vi "Read Discrete Inputs.vi"(8 "error in":errorcluster, 9 "number of inputs":u16, 10 "starting address":u16, 11 "Modbus master in":refnum<class "Modbus Master.lvclass">) -> (0 "error out":errorcluster, 2 "discrete inputs":bool[](array[boolean]), 3 "Modbus master out":refnum<class "Modbus Master.lvclass">)   [LabVIEW 2012, in "Modbus Master.lvclass"]
doc: "Reads <B>number of inputs</B> discrete inputs starting at <B>starting address</B> from the device."
uses:
  Modbus Master.lvclass
  Modbus API.lvclass/Modbus API.ctl
  Modbus Master.lvclass/Modbus Master.ctl
  Transmission Data Unit/Transmission Data Unit.lvclass
  Modbus API.lvclass
  Master Function Definition/Master Function Definition.lvclass
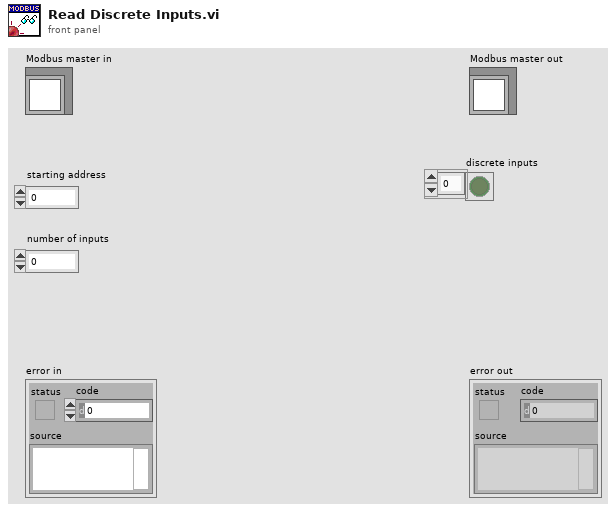
[diagram p1: front panel]
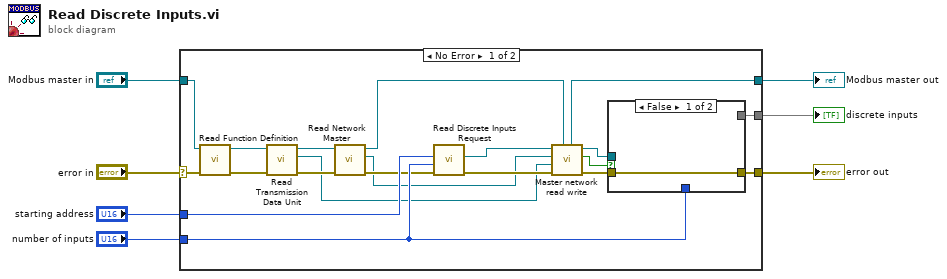
[diagram p0: block diagram]
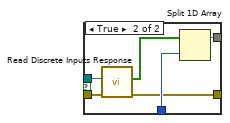
[diagram p2: hidden frame]
diagram:
  n1 = case shown="No Error" "error in" {
    selector: "error in" -> [w14 w35]
    tunnel: "Modbus master in" -> [w11 w36]
    tunnel: [w19 w36] -> w6
    tunnel: [w20 w35] -> w5
    tunnel: [w25 _] -> w3
    tunnel: "number of inputs" -> [w24 _]
    tunnel: "starting address" -> [w26 _]
    frame No Error {
      n2 = call "Read Function Definition.vi"("error in"=w14, "Modbus master in"=w11) -> ("error out"=w17:errorcluster, "Modbus master out"=w16:refnum<class "Modbus Master.lvclass">)  [unwired: 7 in, 1 out]
      n3 = call "Read Transmission Data Unit.vi"("error in"=w17, "Modbus instance in"=w16) -> ("error out"=w15:errorcluster, "transmission data unit"=w10:refnum<class "Transmission Data Unit.lvclass">, "Modbus instance out"=w18:refnum<class "Modbus Master.lvclass">)  [unwired: 7 in]
      n4 = call "Read Network Master.vi"("error in"=w15, "Modbus master in"=w18) -> ("error out"=w13:errorcluster, "network master"=w9:refnum<class "Network Master.lvclass">, "Modbus master out"=w12:refnum<class "Modbus Master.lvclass">)  [unwired: 7 in]
      n5 = call "Read Discrete Inputs Request.vi"("error in"=w13, "Number of inputs"=w24, "starting address"=w26) -> ("error out"=w27:errorcluster, "modbus data unit out"=w22:refnum<class "Modbus Data Unit.lvclass">)  [unwired: 7 in]
      n6 = call "Master network read write.vi"("Modbus master in"=w12, "error in"=w27, "transmission data unit in"=w10, "network master in"=w9, "Modbus data unit in"=w22) -> ("error out"=w23:errorcluster, "PDU Valid?"=w8:bool, "Modbus data unit out"=w21:refnum<class "Modbus Data Unit.lvclass">, "Modbus master out"=w19:refnum<class "Modbus Master.lvclass">)  [unwired: 3 in]
      n7 = case shown="False" w8 {
        tunnel: [_ w33] -> w25
        tunnel: w24 -> [_ w32]
        tunnel: w23 -> [w28 w31]
        tunnel: w21 -> [_ w30]
        tunnel: [w28 w29] -> w20
        frame False {
        }
        frame True {
          n8 = call "Read Discrete Inputs Response.vi"("error in"=w31, "modbus data unit in"=w30) -> ("error out"=w29:errorcluster, "Data"=w34:bool[])  [unwired: 8 in]
          n9 = Split 1D Array(array=w34, index=w32) -> (first subarray=w33:bool[])  [unwired: 1 out]
        }
      }
    }
    frame Error {
    }
  }
  "error out" <- w5
  "Modbus master out" <- w6
  "discrete inputs" <- w3
